vi "Log_TCP.vi"(1 "Data":string, 12 "error in (no error)":errorcluster, 13 "Response? (F: LV Writes)":bool) -> (3 "Data dup":string, 14 "error out":errorcluster)   [LabVIEW 2014]
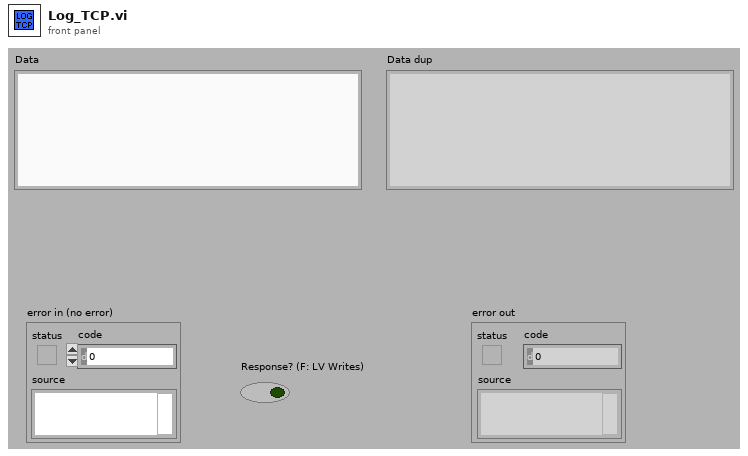
[diagram p1: front panel]
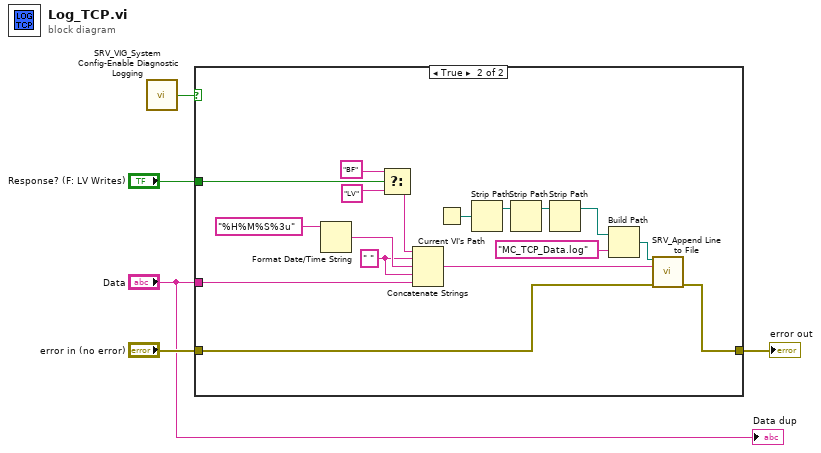
[diagram p0: block diagram]
diagram:
  n1 = call "SRV_VIG_System Config-Enable Diagnostic Logging.vi"() -> ("Enable Diagnostic Log?"=w1:bool)  [unwired: 15 in]
  n2 = case shown="True" w1 {
    tunnel: [w6 w20] -> w5
    tunnel: "error in (no error)" -> [w6 w19]
    tunnel: "Response? (F: LV Writes)" -> [_ w16]
    tunnel: "Data" -> [_ w13]
    frame False {
    }
    frame True {
      w18 = " " ("string")
      n3 = Format Date/Time String(time format string (%c)="%H%M%S%3u") -> (date/time string=w22:string)  [unwired: 2 in]
      n4 = Select(t="BF" ("string"), s=w16, f="LV" ("string")) -> (s? t:f=w14:string)
      n5 = Concatenate Strings(w14, w18, w22, w18, w13) -> (w21:string)
      n6 = Current VI's Path() -> (path=w8:path)
      n7 = Strip Path(path=w8) -> (stripped path=w9:path)  [unwired: 1 out]
      n8 = Strip Path(path=w9) -> (stripped path=w10:path)  [unwired: 1 out]
      n9 = Strip Path(path=w10) -> (stripped path=w7:path)  [unwired: 1 out]
      n10 = Build Path(base path=w7, name or relative path="MC_TCP_Data.log") -> (appended path=w11:path)
      n11 = call "SRV_Append Line to File.vi"("file path"=w11, "Line to Write"=w21, "error in (no error)"=w19) -> ("error out"=w20:errorcluster)  [unwired: 12 in]
    }
  }
  "error out" <- w5
  "Data dup" <- "Data"
